vi "UTIL Clean Up Files.vi"(6 "Delete File":bool, 8 "Error In":errorcluster, 11 "File Path In":path) -> (0 "Error Out":errorcluster, 2 "File Size":i64, 3 "File Path Out":path)   [LabVIEW 2010]
doc: "This VI opens a file, returns its size, and closes (or deletes) it.\n\nInputs:\n File Path In Path\n Delete File Boolean\n Error In\nOutputs:\n File Path Out Passthrough\n Files Size I64\n Error Out"
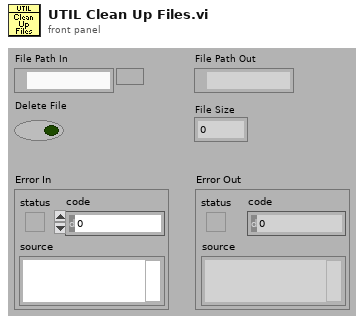
[diagram p1: front panel]
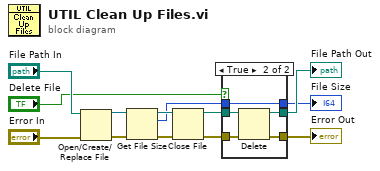
[diagram p0: block diagram]
diagram:
  n1 = Open/Create/Replace File(file path (use dialog)="File Path In", error in="Error In") -> (refnum out=w12:refnum<file>, error out=w13:errorcluster)  [unwired: 4 in, 1 out]
  n2 = Get File Size(file=w12, error in=w13) -> (refnum out=w10:refnum<file>, size (in bytes)=w2:i64, 0:w11:errorcluster)
  n3 = Close File(refnum=w10, error in=w11) -> (path=w8:path, error out=w9:errorcluster)
  n4 = case shown="True" "Delete File" {
    tunnel: w9 -> [w16 w21]
    tunnel: w8 -> [w15 w20]
    tunnel: [w16 w19] -> w6
    tunnel: [w15 w18] -> w5
    tunnel: w2 -> [w14 w17]
    tunnel: [w14 w17] -> w1
    frame False {
    }
    frame True {
      n5 = Delete(path (use dialog)=w20, error in=w21) -> (deleted path=w18:path, error out=w19:errorcluster)  [unwired: 3 in, 1 out]
    }
  }
  "Error Out" <- w6
  "File Size" <- w1
  "File Path Out" <- w5
